vi "configuration.vi"() -> ()   [LabVIEW 2015]
panel:
  in  "Value":i32
  in  "Property":T1(ring)
  in  "FrameRate":string
  out "VideoFormats":string[](array[string])
  in  "VideoNorm":string
  in  "Error In (no error)":errorcluster
  out "Error Out":errorcluster
  out "ICImagingControl Out":refnum<k7>
  in  "VideoFormat":string
  in  "ICImagingControl":refnum<k7>(container)
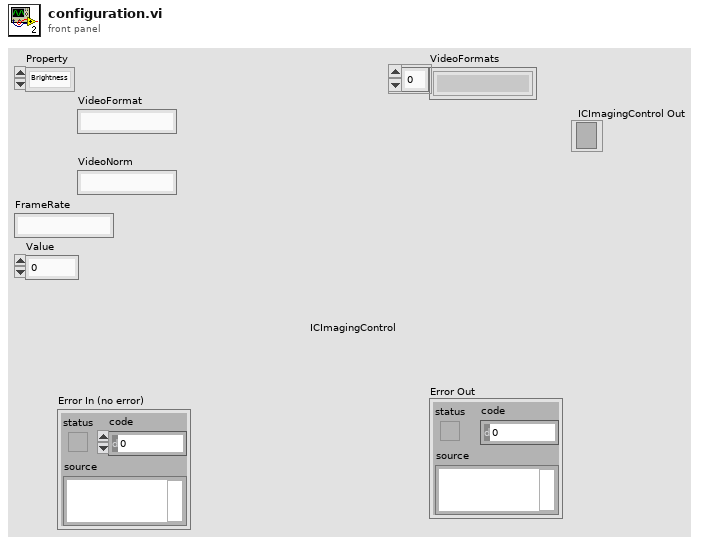
[diagram p1: front panel]
types:
  T1 = enum16{"Brightness", "Color Enable", "Contrast", "Exposure", "Focus", "Gain", "Gamma", "Hue", "Iris", "Pan", "Roll", "Saturation", "Sharpness", "Tilt", "Whitebalance", "Zoom", "Whitebalance Blue", "Whitebalance Red"}
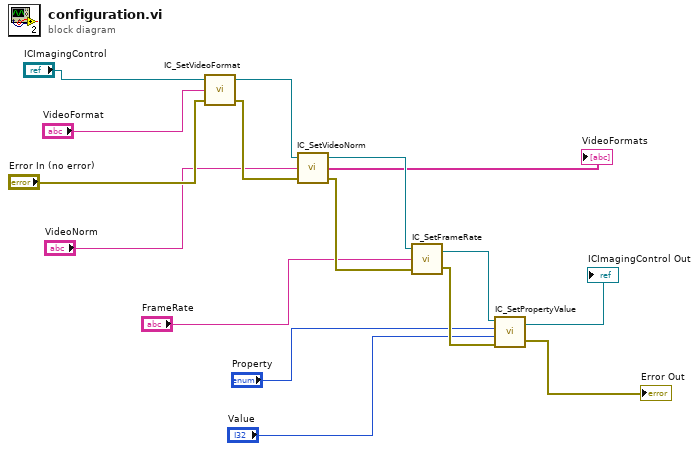
[diagram p0: block diagram]
diagram:
  n1 = call <userlib>:"IC_SetVideoFormat.vi"("Error In (no error)"="Error In (no error)", "VideoFormat"="VideoFormat", "ICImagingControl In"="ICImagingControl") -> ("Error Out"=w15:errorcluster, "ICImagingControl Out"=w11:refnum<k7>)  [unwired: 1 out]
  n2 = call <userlib>:"IC_SetVideoNorm.vi"("Error In (no error)"=w15, "VideoNorm"="VideoNorm", "ICImagingControl In"=w11) -> ("Error Out"=w14:errorcluster, "VideoFormats"=→"VideoFormats":string[], "ICImagingControl Out"=w10:refnum<k7>)
  n3 = call <userlib>:"IC_SetFrameRate.vi"("Error In (no error)"=w14, "FrameRate"="FrameRate", "ICImagingControl In"=w10) -> ("Error Out"=w13:errorcluster, "ICImagingControl Out"=w9:refnum<k7>)
  n4 = call <userlib>:"IC_SetPropertyValue.vi"("Error In (no error)"=w13, "Value"="Value", "Property"="Property", "ICImagingControl In"=w9) -> ("Error Out"=→"Error Out":errorcluster, "ICImagingControl Out"=→"ICImagingControl Out":refnum<k7>)
